vi "Included.vi"(11 "Entity Collection in":refnum<class "Entity Collection.lvclass">) -> (2 "Included":bool)   [LabVIEW 2020, in "Conditu2.lvlib" / "Columns.lvlib" / "Entity Collection.lvclass"]
uses:
  Entity Collection.lvclass
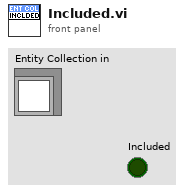
[diagram p1: front panel]
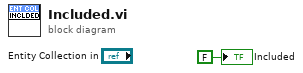
[diagram p0: block diagram]
diagram:
  "Included" <- FALSE ("Included")
